vi "Sort Array with Dublicates.vi"(0 "Clones in":refnum<vi>[](array[refnum])) -> (14 "Clones out":refnum<vi>[](array[refnum]), 15 "Libraries":string[](array[string]))   [LabVIEW 2019]
uses:
  6ffdc9f8-0a2e-443d-8b36-0bf95ddf899b.vi
panel:
  out "Array 2":string[](array[string])
  out "Array":string[](array[string])
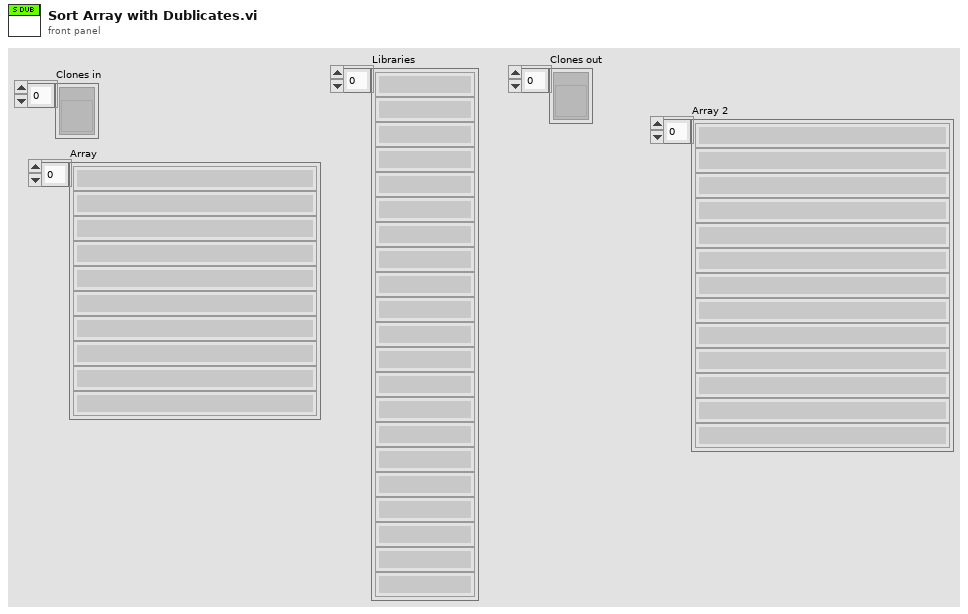
[diagram p1: front panel]
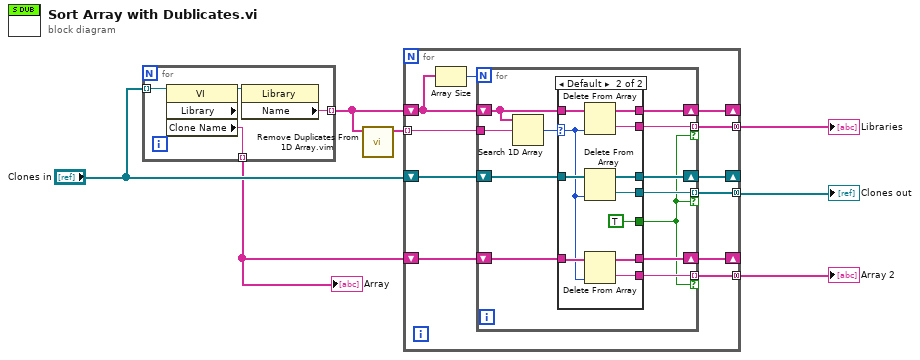
[diagram p0: block diagram]
diagram:
  n1 = for {
    tunnel: "Clones in" -> [w11] mode=indexing
    tunnel: [w9] -> w4 mode=indexing
    tunnel: [w8] -> w2 mode=indexing
    n2 = property class="VI"(reference=w11) -> ("Library"=w10:refnum<vi>, "Clone Name"=w8:string)  [unwired: 1 in, 2 out]
    n3 = property class="Library"(reference=w10) -> ("Name"=w9:string)  [unwired: 1 in, 2 out]
  }
  "Array" <- w2
  n4 = call "Remove Duplicates From 1D Array.vim"("array"=w4) -> ("array with duplicates removed"=w7:string[])  [unwired: 10 in]
  n5 = for {
    tunnel: w7 -> [w22] mode=indexing
    tunnel: [w21] -> w6 mode=concatenating
    shift-right: [w19] -> _
    shift-left: w4 -> [w18]
    shift-right: [w16] -> _
    shift-left: "Clones in" -> [w17]
    tunnel: [w15] -> w5 mode=concatenating
    shift-right: [w13] -> _
    shift-left: w2 -> [w14]
    tunnel: [w12] -> w1 mode=concatenating
    n6 = Array Size(array=w18) -> (size(s)=w20:i32)
    n7 = for {
      N: w20 -> [_]
      tunnel: w22 -> [w34]
      tunnel: [w32] -> w21 mode=indexing if=w23
      shift-right: [w33] -> w19
      shift-left: w18 -> [w31]
      shift-right: [w28] -> w16
      shift-left: w17 -> [w29]
      tunnel: [w27] -> w15 mode=indexing if=w23
      shift-right: [w26] -> w13
      shift-left: w14 -> [w25]
      tunnel: [w24] -> w12 mode=indexing if=w23
      n8 = Search 1D Array(1D array=w31, element=w34) -> (index of element=w30:i32)  [unwired: 1 in]
      n9 = case shown="Default" w30 {
        selector: w30 -> [_ w38]
        tunnel: w31 -> [w37 w48]
        tunnel: [w37 w47] -> w33
        tunnel: [_ w46] -> w32
        tunnel: [_ TRUE] -> w23
        tunnel: w29 -> [w36 w44]
        tunnel: [w36 w43] -> w28
        tunnel: [_ w42] -> w27
        tunnel: [w35 w41] -> w26
        tunnel: w25 -> [w35 w40]
        tunnel: [_ w39] -> w24
        frame -1 {
        }
        frame Default {
          n10 = Delete From Array(array=w48, index=w38) -> (deleted portion=w46:string, array with subset deleted=w47:string[])  [unwired: 1 in]
          n11 = Delete From Array(array=w44, index=w38) -> (deleted portion=w42:refnum<vi>, array with subset deleted=w43:refnum<vi>[])  [unwired: 1 in]
          n12 = Delete From Array(array=w40, index=w38) -> (deleted portion=w39:string, array with subset deleted=w41:string[])  [unwired: 1 in]
        }
      }
    }
  }
  "Libraries" <- w6
  "Clones out" <- w5
  "Array 2" <- w1
